vi "Generate Task.vi"(8 "error in (no error)":errorcluster, 10 "Task Factory MSG In":refnum<class "Task Factory MSG.lvclass">, 11 "Task Factory in":refnum<class "Task Factory.lvclass">) -> (0 "error out":errorcluster, 3 "Task Factory out":refnum<class "Task Factory.lvclass">)   [LabVIEW 2024, in "Task Factory.lvclass"]
uses:
  Task Factory.lvclass
  Task Factory MSG/Task Factory MSG.lvclass
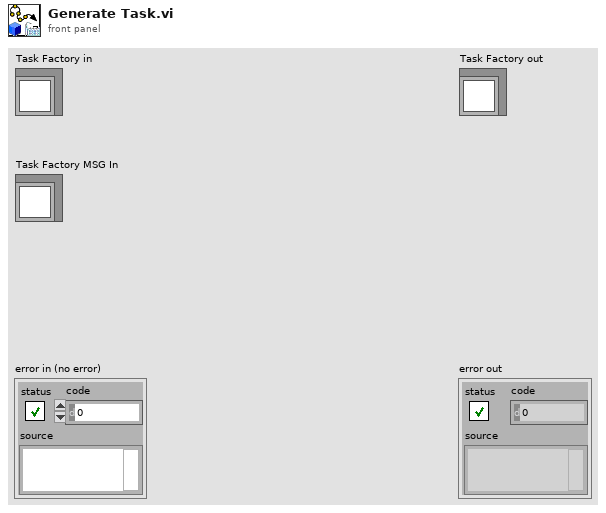
[diagram p1: front panel]
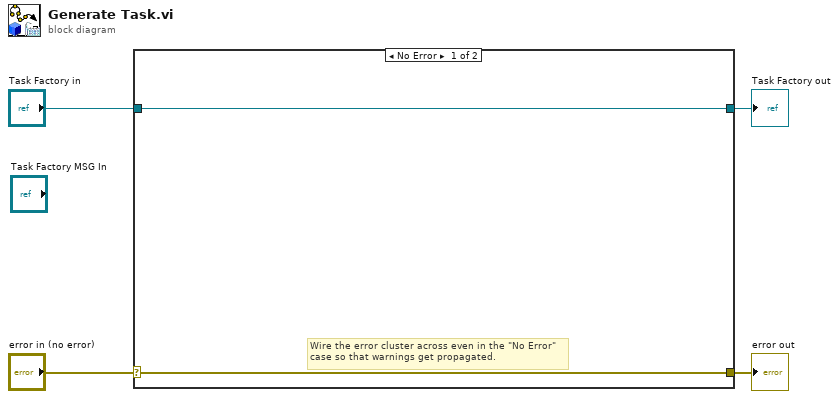
[diagram p0: block diagram]
diagram:
  n1 = case shown="No Error" "error in (no error)" {
    selector: "error in (no error)" -> [w5 w8]
    tunnel: [w5 w8] -> w3
    tunnel: [w6 w7] -> w1
    tunnel: "Task Factory in" -> [w6 w7]
    frame No Error {
      # "Wire the error cluster across even in the \"No Error\"\ncase so that warnings get propagated."
    }
    frame Error {
    }
  }
  "error out" <- w3
  "Task Factory out" <- w1
